vi "Draw Current Position Marker.vi"(1 "Current Location":i32, 2 "Array 2":T1[](array[typedef])) -> (0 "Array":T1[](array[typedef]))   [LabVIEW 2012, in "Waveform Control.xctl"]
doc: "Generates a waveform that is NaN apart from the one point at the given index position. The Y value of this point is the same as the corresponding point in the first waveform of the array input,"
uses:
  Waveform Control.xctl
  Controls/Data.ctl
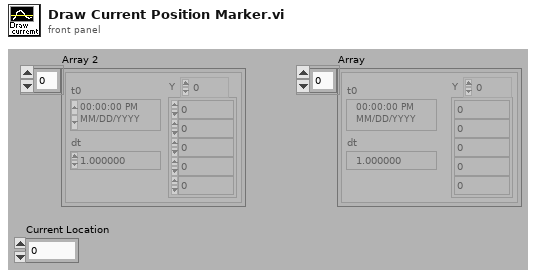
[diagram p1: front panel]
types:
  T1 = typedef "Waveform Control.xctl/Data.ctl" = waveform(dbl)
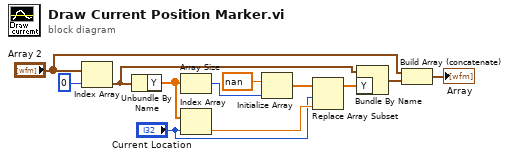
[diagram p0: block diagram]
diagram:
  n1 = Index Array(array="Array 2", index=0) -> (element=w9:T1)
  n2 = Unbundle By Name(w9) -> ("Y"=w6:dbl[])
  n3 = Array Size(array=w6) -> (size(s)=w2:i32)
  n4 = Index Array(array=w6, index="Current Location") -> (element=w7:dbl)
  n5 = Initialize Array(nan ("element"), w2) -> (w4:dbl[])
  n6 = Replace Array Subset(array=w4, new element=w7, index="Current Location") -> (w8:dbl[])
  n7 = Bundle By Name(cluster=w9, "Y"=w8) -> (w11:T1)
  n8 = Build Array (concatenate)("Array 2", w11) -> (→"Array":T1[])
